vi "getClaseReceta.vi"(6 "error in":errorcluster, 9 "claseReceta in":refnum<class "claseReceta.lvclass">) -> (0 "error out":errorcluster, 2 "dataReading":T1, 3 "claseReceta out":refnum<class "claseReceta.lvclass">)   [LabVIEW 2014, in "claseReceta.lvclass"]
uses:
  claseReceta.lvclass
  claseReceta.lvclass/claseReceta.ctl
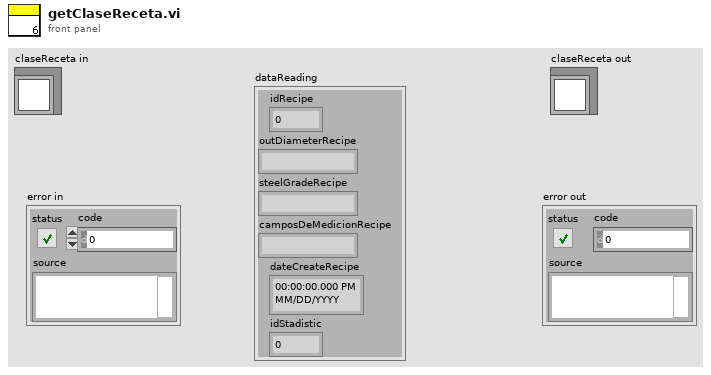
[diagram p1: front panel]
types:
  T1 = cluster{"idRecipe":dbl, "outDiameterRecipe":string, "steelGradeRecipe":string, "camposDeMedicionRecipe":string, "dateCreateRecipe":timestamp, "idStadistic":dbl}
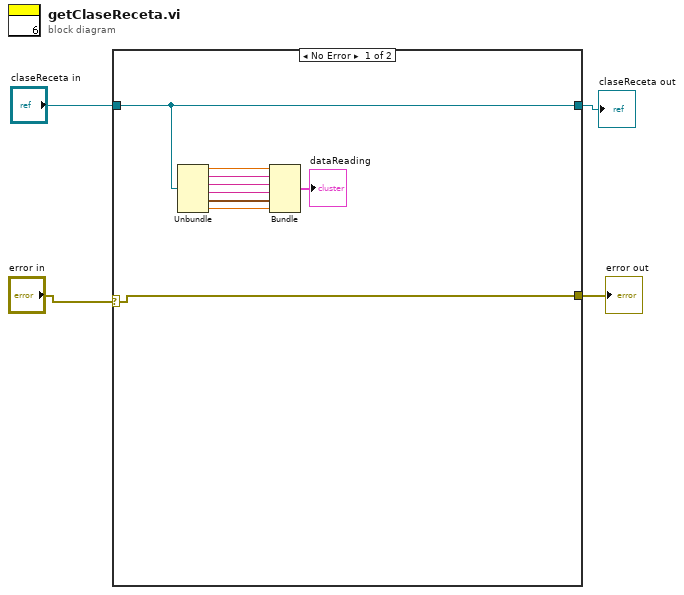
[diagram p0: block diagram]
diagram:
  n1 = case shown="No Error" "error in" {
    selector: "error in" -> [w13 w15]
    tunnel: [w13 w15] -> w3
    tunnel: "claseReceta in" -> [w12 w14]
    tunnel: [w12 w14] -> w1
    frame No Error {
      n2 = Unbundle(w12) -> (w11:dbl, w10:string, w9:string, w8:string, w7:timestamp, w6:dbl)
      n3 = Bundle("idRecipe"=w11, "outDiameterRecipe"=w10, "steelGradeRecipe"=w9, "camposDeMedicionRecipe"=w8, "dateCreateRecipe"=w7, "idStadistic"=w6) -> (→"dataReading":T1)  [unwired: 1 in]
    }
    frame Error {
    }
  }
  "claseReceta out" <- w1
  "error out" <- w3
